vi "Return Timeout Error.vi"(7 "error source vi name":string, 8 "error in (no error)":errorcluster, 10 "iteration":u64=1, 11 "Transfer Group in":refnum<class "Transfer Group.lvclass">) -> (0 "error out":errorcluster, 3 "Transfer Group out":refnum<class "Transfer Group.lvclass">)   [LabVIEW 2017, in "DSF Core.lvlib" / "Transfer Group.lvclass"]
uses:
  Transfer Group.lvclass
  Errors.ctl
  Transfer Group.lvclass/Transfer Group.ctl
  <vilib>/NI/Memory Manager/VIs/New Error Cluster (512B).vi
  <vilib>/NI/Memory Manager/VIs/Write Numeric Scalar to Source (Base10 I32).vi
  <vilib>/NI/Memory Manager/VIs/Write Numeric Scalar to Source (Base10 U64).vi
  Framework/Engine Library Name.vi
  Framework/Framework.lvclass
  <vilib>/NI/Memory Manager/Static Errors.lvlib
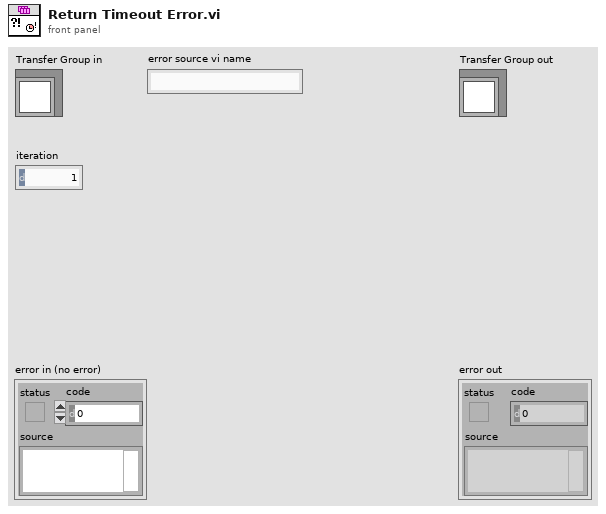
[diagram p1: front panel]
types:
  T1 = typedef "DSF Core.lvlib/Transfer Group.lvclass/Errors.ctl" = enum16{"Return Timeout", "Invalid Iteration"}
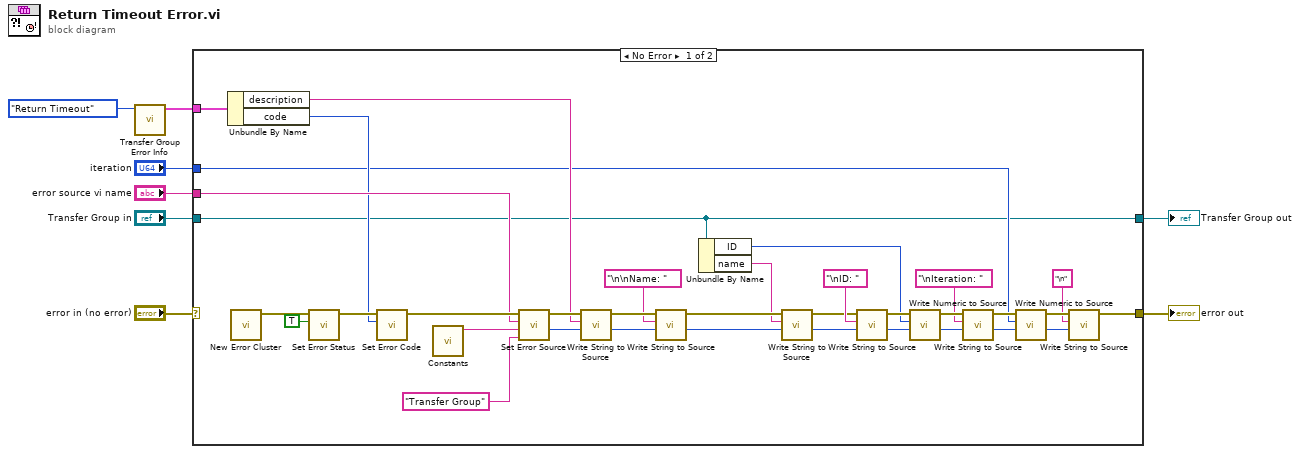
[diagram p0: block diagram]
diagram:
  n1 = call "Transfer Group Error Info.vi"("errors"=Errors."Return Timeout") -> ("error info"=w1:cluster{"code":i32, "description":string})  [unwired: 10 in]
  n2 = case shown="No Error" "error in (no error)" {
    selector: "error in (no error)" -> [_ w44]
    tunnel: [w31 w44] -> w7
    tunnel: [w12 w45] -> w6
    tunnel: "Transfer Group in" -> [w12 w45]
    tunnel: "error source vi name" -> [w35 _]
    tunnel: "iteration" -> [w19 _]
    tunnel: w1 -> [w27 _]
    frame No Error {
      n3 = Unbundle By Name(w27) -> ("description"=w22:string, "code"=w26:i32)
      n4 = call-poly <vilib>:"New Error Cluster.vi"() -> ("error out"=w43:errorcluster)  [unwired: 10 in, 1 out]
      n5 = call <vilib>:"Set Error Status.vi"("status (T)"=TRUE, "error in"=w43) -> ("error out"=w42:errorcluster)  [unwired: 9 in]
      n6 = call <vilib>:"Set Error Code.vi"("code"=w26, "error in"=w42) -> ("error out"=w41:errorcluster)  [unwired: 9 in]
      n7 = call-poly "Constants.vi"() -> ("Engine Library Name"=w40:string)  [unwired: 11 in]
      n8 = call <vilib>:"Set Error Source.vi"("class name (\"\")"="Transfer Group" ("Engine Library Name"), "library name (\"\")"=w40, "vi name"=w35, "error in"=w41) -> ("initial offset"=w24:i32, "error out"=w25:errorcluster)  [unwired: 6 in]
      n9 = call <vilib>:"Write String to Source.vi"("offset"=w24, "string"=w22, "error in"=w25) -> ("new offset"=w14:i32, "error out"=w15:errorcluster)  [unwired: 7 in]
      n10 = call <vilib>:"Write String to Source.vi"("offset"=w14, "string"="\n\nName: ", "error in"=w15) -> ("new offset"=w10:i32, "error out"=w11:errorcluster)  [unwired: 7 in]
      n11 = Unbundle By Name(w12) -> ("ID"=w18:i32, "name"=w9:string)
      n12 = call <vilib>:"Write String to Source.vi"("offset"=w10, "string"=w9, "error in"=w11) -> ("new offset"=w17:i32, "error out"=w16:errorcluster)  [unwired: 7 in]
      n13 = call <vilib>:"Write String to Source.vi"("offset"=w17, "string"="\nID: ", "error in"=w16) -> ("new offset"=w38:i32, "error out"=w39:errorcluster)  [unwired: 7 in]
      n14 = call-poly <vilib>:"Write Numeric to Source.vi"("offset"=w38, "value"=w18, "error in"=w39) -> ("new offset"=w36:i32, "error out"=w37:errorcluster)  [unwired: 7 in]
      n15 = call <vilib>:"Write String to Source.vi"("offset"=w36, "string"="\nIteration: ", "error in"=w37) -> ("new offset"=w33:i32, "error out"=w34:errorcluster)  [unwired: 7 in]
      n16 = call-poly <vilib>:"Write Numeric to Source.vi"("offset"=w33, "value"=w19, "error in"=w34) -> ("new offset"=w30:i32, "error out"=w32:errorcluster)  [unwired: 7 in]
      n17 = call <vilib>:"Write String to Source.vi"("offset"=w30, "string"="\n", "error in"=w32) -> ("error out"=w31:errorcluster)  [unwired: 7 in, 1 out]
    }
    frame Error {
      # "Incoming error. Pass through."
    }
  }
  "error out" <- w7
  "Transfer Group out" <- w6
